vi "Control Ackermann PP.vi"(0 "Setpoints":dbl[](array[numeric]), 5 "state x(k)":dbl[](array[numeric]), 9 "State-Space Model":T2 {"Transport Delay" format="%.2f"; "D" format="%#.2g"; "C" format="%#.2g"; "B" format="%#.2g"; "A" format="%#.2g"; "properties"."Sampling Time" format="%#.6p"; "properties"."Output Delays" format="%.4f"; "properties"."Input Delays" format="%.4f"}, 11 "Real":dbl(knob)=-3.4076115316471642 scale=0.0..-22.0 scale format="%#_4g", 12 "Imaginary":dbl(knob)=-10.013861291935129 scale=0.0..-20.0 scale format="%#_4g") -> (1 "Actual Poles":cdb[](array[numeric])=[-4.9512521676495505+0.0i, -3.4076115316471447-10.013861291935113i, -3.4076115316471447+10.013861291935113i] format="%.2f", 3 "Desired Poles":cdb[](array[numeric])=[-4.951252167649562+0.0i, -3.4076115316471642-10.013861291935129i, -3.4076115316471642+10.013861291935129i] format="%.2f", 4 "u(k)":dbl format="%.2f", 6 "Controller Action":dbl format="%#.2g", 8 "State Trajectory Graph":cluster{"time":dbl[], dbl[]}[](graph), 10 "Closed-Loop Step Response":cluster{"time":dbl[], dbl[]}[](graph), 13 "Gain":dbl[](array[numeric]) format="%.3f", 14 "Time Response Parametric Data":T1={"Rise Time (s)"=[[0.0, 0.0], [0.0, 0.0]], "Peak Time (s)"=[[16.01539885840777, 17.159355919722614], [7.372167728473419, 117.70047097528251]], "Settling Time (s)"=[[0.0, 0.0], [0.0, 0.0]], "Overshoot (%)"=[[2.6933680524159342, 1.5395749934973058], [324.8704022191171, -0.0007732741527544107]], "Steady-State Gain"=[[0.0, 0.0], [0.0, 0.0]], "Peak Value"=[[0.0, 0.0], [0.0, 0.0]]}, 15 "error out":errorcluster)   [LabVIEW 2017]
uses:
  <vilib>/addons/Control Design/_Model Construction/Model Typedefs.llb/CD State Space Model (MIMO).ctl
  <vilib>/addons/Control Design/_Model Construction/Model Typedefs.llb/CD General Elements.ctl
  <vilib>/addons/Control Design/_Model Construction/Data Typedefs.llb/CD Parametric Time Response Data.ctl
  <vilib>/Analysis/baseanly.llb/Real Dot Product.vi
  <vilib>/addons/Control Design/_Implementation/CD State Feedback Controller (Single Output).vi
  <vilib>/Analysis/NI_AALBase.lvlib
  <vilib>/addons/Control Design/_Implementation/NI_CD_Implementation.lvlib
  <vilib>/addons/Control Design/_Model Construction/NI_LinSys_Model Typedefs.lvlib
  <vilib>/addons/Control Design/_Model Construction/NI_LinSys_Data Typedefs.lvlib
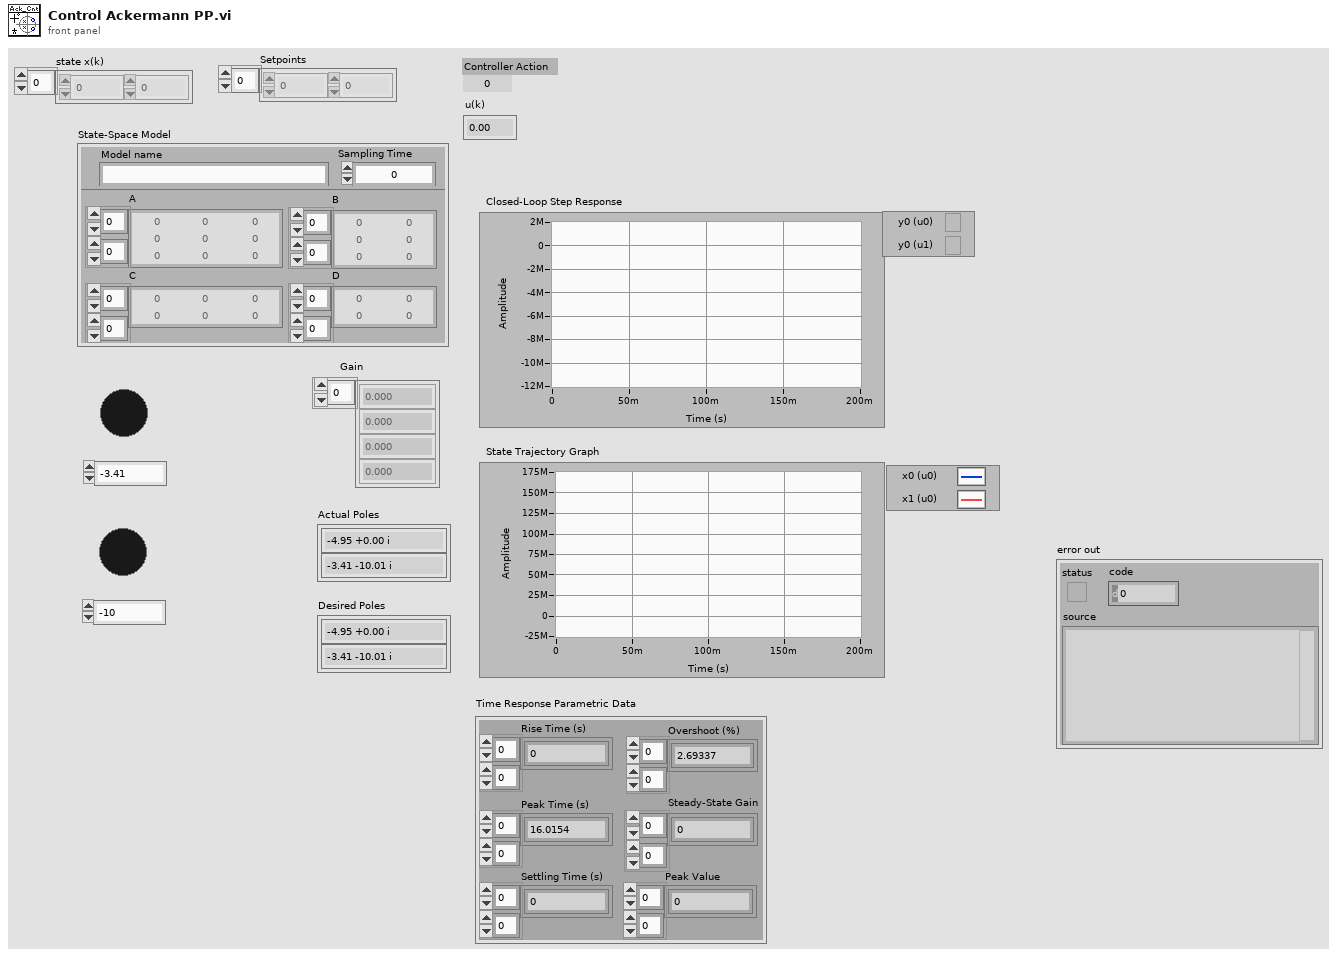
[diagram p1: front panel]
types:
  T1 = typedef "NI_LinSys_Data Typedefs.lvlib/CD Parametric Time Response Data.ctl" = cluster{"Rise Time (s)":dbl[][], "Peak Time (s)":dbl[][], "Settling Time (s)":dbl[][], "Overshoot (%)":dbl[][], "Steady-State Gain":dbl[][], "Peak Value":dbl[][]}
  T2 = typedef "NI_LinSys_Model Typedefs.lvlib/CD State Space Model (MIMO).ctl" = cluster{"properties":T3, "A":dbl[][], "B":dbl[][], "C":dbl[][], "D":dbl[][], "StateNames":string[], "Transport Delay":dbl[][]}
  T3 = typedef "NI_LinSys_Model Typedefs.lvlib/CD General Elements.ctl" = cluster{"Model name":string, "Input names":string[], "Output names":string[], "Input Delays":dbl[], "Output Delays":dbl[], "Sampling Time":dbl, "Notes":string}
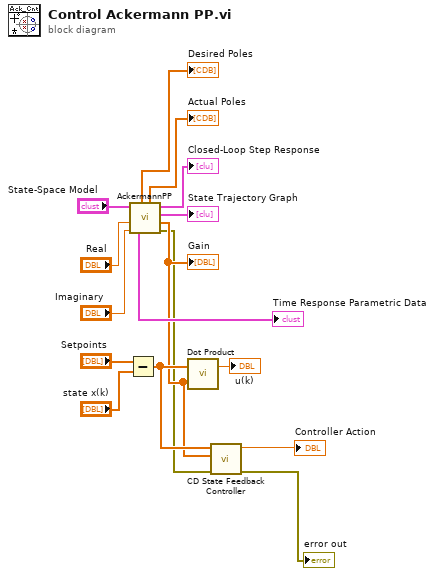
[diagram p0: block diagram]
diagram:
  n1 = Subtract ("Subtract.vi")(x="Setpoints", y="state x(k)") -> (x-y=w6:dbl[])
  n2 = call "AckermannPP.vi"("Imaginary"="Imaginary", "Real"="Real", "State-Space Model"="State-Space Model") -> ("error out"=w2:errorcluster, "Gain"=w3:dbl[], "State Trajectory Graph"=→"State Trajectory Graph":cluster{"time":dbl[], dbl[]}[], "Closed-Loop Step Response"=→"Closed-Loop Step Response":cluster{"time":dbl[], dbl[]}[], "Actual Poles"=→"Actual Poles":cdb[], "Time Response Parametric Data"=→"Time Response Parametric Data":T1, "Desired Poles"=→"Desired Poles":cdb[])  [unwired: 1 in]
  "Gain" <- w3
  n3 = call-poly <vilib>:"Dot Product.vi"("Y Vector"=w3, "X Vector"=w6) -> ("X * Y"=→"u(k)":dbl)  [unwired: 1 out]
  n4 = call-poly <vilib>:"CD State Feedback Controller.vi"("error in (no error)"=w2, "Controller Gain"=w3, "States"=w6) -> ("error out"=→"error out":errorcluster, "Controller Action"=→"Controller Action":dbl)  [unwired: 7 in]
